vi "Send Fetch Min Max Waveform [MmW].vi"(7 "Message Priority (Normal)":T1=enum."Normal", 8 "error in (no error)":errorcluster, 9 "waveform size (0)":i32=1000, 10 "channel name (\"CHANNEL1\")":string="CHANNEL1", 11 "Message Enqueuer":refnum<class "Message Enqueuer.lvclass">) -> (0 "error out":errorcluster, 3 "Message Enqueuer out":refnum<class "Message Enqueuer.lvclass">)   [LabVIEW 2015, in "CS++Scope.lvlib" / "Fetch Min Max Waveform [MmW] Msg.lvclass"]
doc: "Sends the <B>CS++Scope.lvlib:Fetch Min Max Waveform [MmW] Msg.lvclass</B> message.\n\n<B>CS++Scope.lvlib:CS++Scope.lvclass:Fetch Min Max Waveform [MmW].vi</B> Description:\n\nThis VI returns the minimum and maximum waveforms that the oscilloscope acquires for the channel you specify. If the channel is not enabled for the acquisition, this VI returns IVISCOPE_ERROR_CHANNEL_NOT_ENABLED (0xBFFA2001)error.\nThe waveforms are from an acquisition that you previously initiated. Use this VI to fetch waveforms when you set the acquisition type to IVISCOPE_VAL_PEAK_DETECT or IVISCOPE_VAL_ENVELOPE. If the acquisition type is not one of the listed types, the VI returns the IVISCOPE_ERROR_INVALID_ACQ_TYPE (0xBFFA2004) error.\n\nUse the IviScope Initiate Acquisition VI to start an acquisition on the channels that you enable with the IviScope Configure Channel VI. The oscilloscope acquires the min/max waveforms for the enabled channels concurrently. You use the IviScope Acquisition Status VI to determine when the acquisition is complete. You must call this VI separately for each enabled channel to obtain the min/max waveforms.\nYou can call the IviScope Read Min Max Waveform [MmW] VI instead of the IviScope Initiate Acquisition VI. The IviScope Read Min Max Waveform [MmW] VI starts an acquisition on all enabled channels, waits for the acquisition to complete, and returns the min/max waveforms for the channel you specify. You call this VI to obtain the min/max waveforms for each of the remaining channels.\n\nNotes:\n(1) After this VI executes, each element in the Min Waveform Array and Max Waveform Array parameters is either a voltage or a value indicating that the oscilloscope could not sample a voltage.\n\n(2) You configure the interpolation method the oscilloscope uses with the IviScope Is Invalid Waveform Element VI. If you disable interpolation, the oscilloscope does not interpolate points in the waveform. If the oscilloscope cannot sample a value for a point in the waveform, the driver sets the corresponding element in the Waveform Array to an IEEE defined NaN (Not a Number) value and the VI returns IVISCOPE_WARN_INVALID_WFM_ELEMENT (0x3FFA2001). \n\n(3) You can test a waveform value for an invalid value condition by calling the IviScope Is Invalid Waveform Element VI.\n\n(4) This VI does not check the instrument status. Typically, you call this VI only in a sequence of calls to other low-level driver VIs. The sequence performs one operation. You use the low-level VIs to optimize one or more aspects of interaction with the instrument. If you want to check the instrument status, call the IviScope Error-Query VI at the conclusion of the sequence.\n\n(5) The class driver returns a simulated minimum and maximum waveform when this VI is called and the IviScope>>Inherent IVI Settings>>User Options>>Simulate property is set to TRUE and the IviScope>>Inherent IVI Settings>>User Options>>Use Specific Simulation property is set to FALSE. For information on how to configure a simulated waveform, refer to the online help manual.\n\n(6) This VI is part of the IviScopeMinMaxWaveform [MmW] extension group."
uses:
  Fetch Min Max Waveform [MmW] Msg.lvclass
  <vilib>/ActorFramework/Message Enqueuer/Message Enqueuer.lvclass
  <vilib>/ActorFramework/Message Enqueuer/Message Priority.ctl
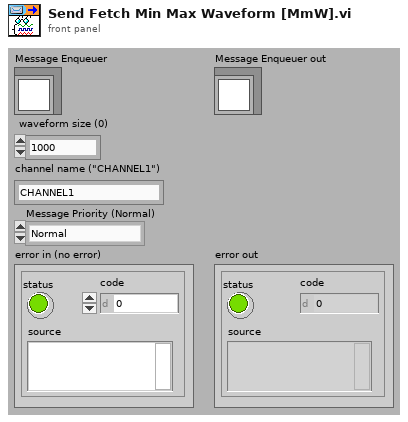
[diagram p1: front panel]
types:
  T1 = typedef "Actor Framework.lvlib/Message Enqueuer.lvclass/Message Priority.ctl" = enum16{"Low", "Normal", "High"}
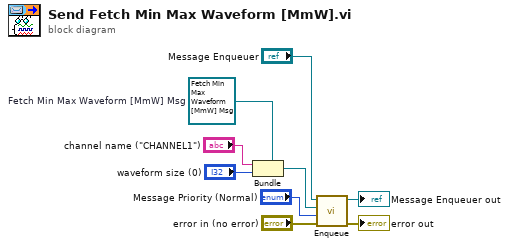
[diagram p0: block diagram]
diagram:
  w3 = refnum<class "Fetch Min Max Waveform [MmW] Msg.lvclass"> refnum  # Fetch Min Max Waveform [MmW] Msg
  n1 = Bundle(cluster=w3, "channel name (\"CHANNEL1\")", "waveform size (0)") -> (w6:refnum<class "Fetch Min Max Waveform [MmW] Msg.lvclass">)
  n2 = call <vilib>:"Enqueue.vi"("error in (no error)"="error in (no error)", "Message Priority (Normal)"="Message Priority (Normal)", "Message"=w6, "Message Enqueuer in"="Message Enqueuer") -> ("error out"=→"error out":errorcluster, "Message Enqueuer out"=→"Message Enqueuer out":refnum<class "Message Enqueuer.lvclass">)  [unwired: 6 in]
